vi "AdvFilter-Apply.vi"(0 "Filter":T1 {"Stages"."IIR Filter"."Forward Coefficients" format="%.4f"; "Stages"."IIR Filter"."Reverse Coefficients" format="%.4f"}, 7 "X":dbl[](array[numeric]), 11 "error in (no error)":errorcluster) -> (4 "Filter out":T1 {"Stages"."IIR Filter"."Forward Coefficients" format="%.4f"; "Stages"."IIR Filter"."Reverse Coefficients" format="%.4f"}, 8 "Filtered X":dbl[](array[numeric]), 15 "error out":errorcluster)   [LabVIEW 2020]
uses:
  Controls/Advanced Filter XCtl/Filter Data.ctl
  Filter-Bandwidth Units.ctl
  <vilib>/Analysis/3filter.llb/IIR Cascade Filter with I.C. (DBL).vi
  <vilib>/Analysis/NI_AALBase.lvlib
  Controls/Advanced Filter XCtl/Advanced Filter XCtl.xctl
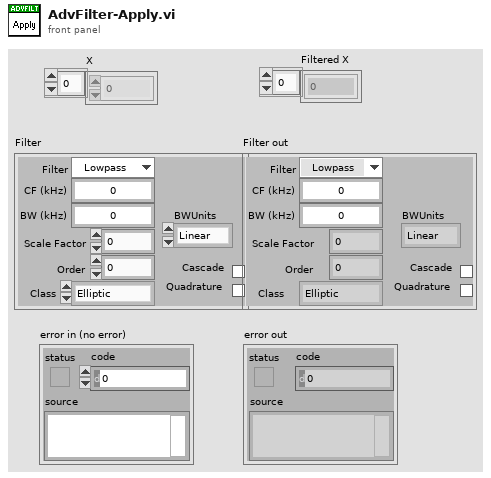
[diagram p1: front panel]
types:
  T1 = typedef "Advanced Filter XCtl.xctl/Filter Data.ctl" = cluster{"Type":enum16{"Lowpass", "Highpass", "Bandpass", "Bandstop", "OFF"}, "CF (kHz)":dbl, "BW (kHz)":dbl, "Cascade":bool, "Quadrature":bool, "Scale Factor":dbl, "Stages":cluster{"IIR Filter":cluster{"filter structure":enum32{"IIR 2nd Order", "IIR 4th Order"}, "Reverse Coefficients":dbl[], "Forward Coefficients":dbl[]}, "State":dbl[]}[], "Class":enum16{"Elliptic", "Butterworth"}, "Order":i32, "BWUnits":T2}
  T2 = typedef "Filter-Bandwidth Units.ctl" = enum16{"Linear", "Octaves", "Min-Max"}
  T3 = enum16{"Lowpass", "Highpass", "Bandpass", "Bandstop", "OFF"}
  T4 = cluster{"IIR Filter":cluster{"filter structure":enum32{"IIR 2nd Order", "IIR 4th Order"}, "Reverse Coefficients":dbl[], "Forward Coefficients":dbl[]}, "State":dbl[]}[]
  T5 = cluster{"filter structure":enum32{"IIR 2nd Order", "IIR 4th Order"}, "Reverse Coefficients":dbl[], "Forward Coefficients":dbl[]}
  T6 = cluster{"IIR Filter":cluster{"filter structure":enum32{"IIR 2nd Order", "IIR 4th Order"}, "Reverse Coefficients":dbl[], "Forward Coefficients":dbl[]}, "State":dbl[]}
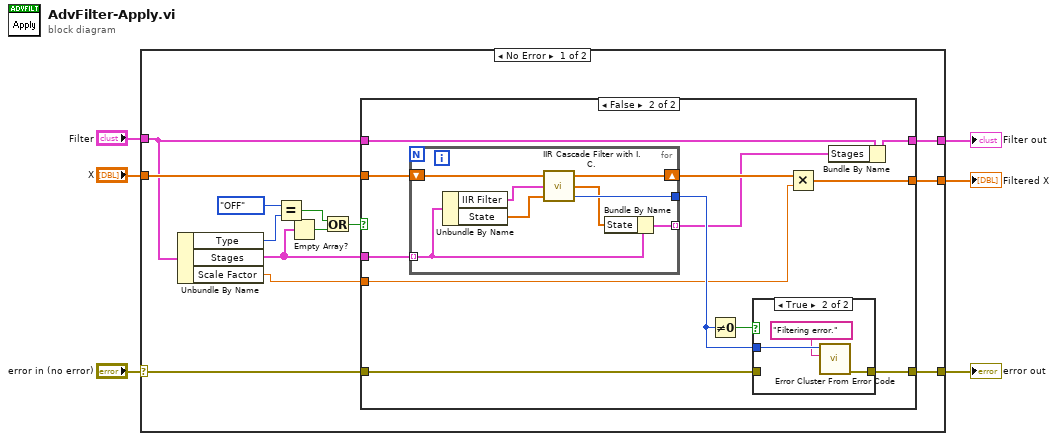
[diagram p0: block diagram]
diagram:
  n1 = case shown="No Error" "error in (no error)" {
    selector: "error in (no error)" -> [w16 w49]
    tunnel: "X" -> [w19 w48]
    tunnel: "Filter" -> [w18 w47]
    tunnel: [w17 w49] -> w5
    tunnel: [w15 w48] -> w3
    tunnel: [w14 w47] -> w2
    frame No Error {
      n2 = Unbundle By Name(w18) -> ("Type"=w12:T3, "Stages"=w9:T4, "Scale Factor"=w13:dbl)
      n3 = Equal?(x=T3."OFF", y=w12) -> (x = y?=w10:bool)
      n4 = Empty Array?(array=w9) -> (empty?=w8:bool)
      n5 = Or(x=w10, y=w8) -> (x .or. y?=w7:bool)
      n6 = case shown="False" w7 {
        tunnel: w19 -> [w22 w34]
        tunnel: w9 -> [_ w23]
        tunnel: w18 -> [w20 w26]
        tunnel: [w21 w32] -> w17
        tunnel: w16 -> [w21 w30]
        tunnel: [w22 w27] -> w15
        tunnel: [w20 w24] -> w14
        tunnel: w13 -> [_ w28]
        frame True {
        }
        frame False {
          n7 = for {
            tunnel: [w41] -> w31
            shift-right: [w40] -> w29
            shift-left: w34 -> [w42]
            tunnel: w23 -> [w38] mode=indexing
            tunnel: [w36] -> w25 mode=indexing
            n8 = Unbundle By Name(w38) -> ("IIR Filter"=w39:T5, "State"=w35:dbl[])
            n9 = call-poly <vilib>:"IIR Cascade Filter with I.C..vi"("Initial Filter State"=w35, "IIR Filter Cluster"=w39, "X"=w42) -> ("error"=w41:i32, "Final Filter State"=w37:dbl[], "Filtered X"=w40:dbl[])
            n10 = Bundle By Name(cluster=w38, "State"=w37) -> (w36:T6)
          }
          n11 = Not Equal To 0?(x=w31) -> (x != 0?=w33:bool)
          n12 = case shown="True" w33 {
            tunnel: w30 -> [w43 _]
            tunnel: [w43 w45] -> w32
            tunnel: w31 -> [_ w46]
            frame False {
            }
            frame True {
              n13 = call <vilib>:"Error Cluster From Error Code.vi"("error message (\"\")"="Filtering error." ("error message (\"\")"), "error code (0)"=w46) -> ("error out"=w45:errorcluster)  [unwired: 7 in]
            }
          }
          n14 = Multiply(x=w29, y=w28) -> (x*y=w27:dbl[])
          n15 = Bundle By Name(cluster=w26, "Stages"=w25) -> (w24:T1)
        }
      }
    }
    frame Error {
    }
  }
  "error out" <- w5
  "Filtered X" <- w3
  "Filter out" <- w2
